vi "Retrieve trace.vi"(5 "max points":i32, 6 "error in (no error)":errorcluster, 7 "Data.PG in":refnum<class "Data.PG.lvclass">, 8 "Column path":string, 9 "Table path":string, 10 "End":timestamp, 11 "Start":timestamp) -> (0 "error out":errorcluster, 2 "Trace":cluster{timestamp[], dbl[]}, 3 "Data.PG out":refnum<class "Data.PG.lvclass">)   [LabVIEW 2020, in "Data.PG.lvclass"]
uses:
  Data.PG.lvclass
  <vilib>/Utility/error.llb/Error Cluster From Error Code.vi
  <vilib>/ErrorRing/Error Ring.xnode
panel:
  out "resulting string":string
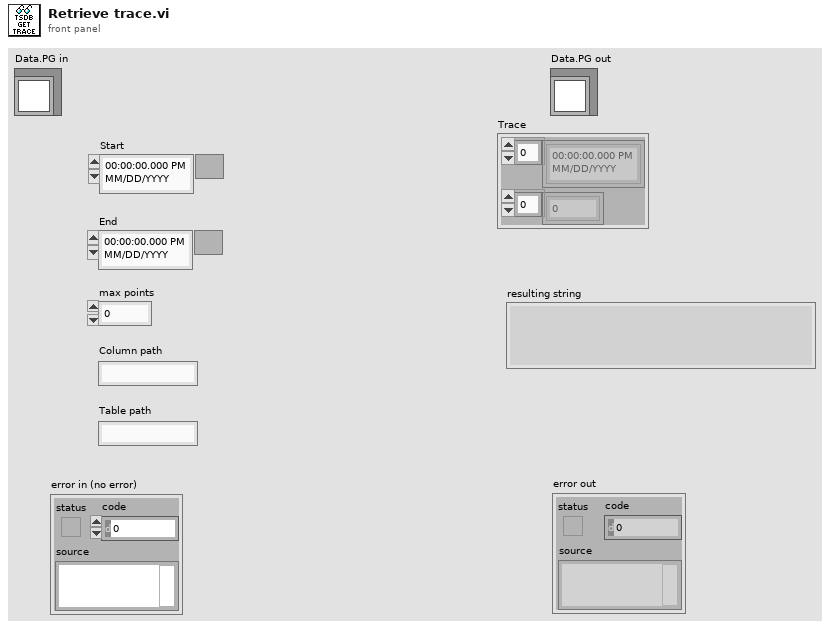
[diagram p1: front panel]
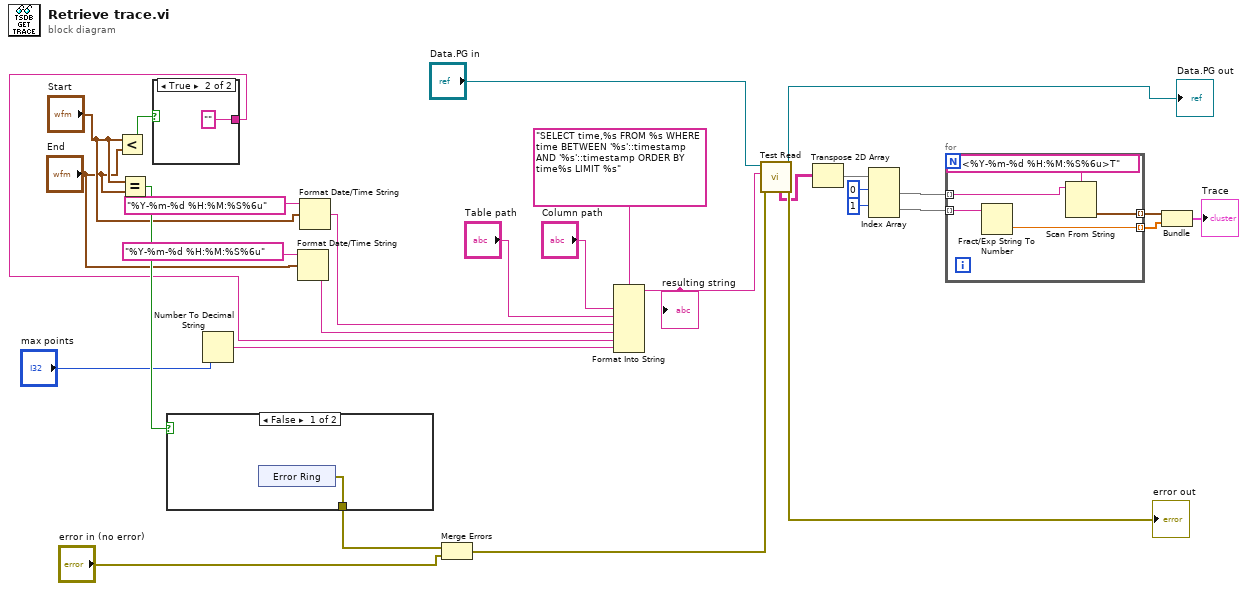
[diagram p0: block diagram]
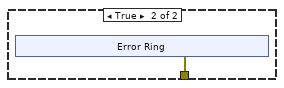
[diagram p2: hidden frame]
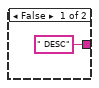
[diagram p3: hidden frame]
diagram:
  n1 = Less?(x="Start", y="End") -> (x < y?=w27:bool)
  n2 = Equal?(x="Start", y="End") -> (x = y?=w26:bool)
  n3 = case shown="True" w27 {
    tunnel: [" DESC" ""] -> w1
    frame False {
    }
    frame True {
    }
  }
  n4 = case shown="False" w26 {
    tunnel: [w33 w35] -> w25
    frame False {
      n5 = xnode "Error Ring"() -> ("error out"=w33:errorcluster)
    }
    frame True {
      n6 = xnode "Error Ring"() -> ("error out"=w35:errorcluster)
    }
  }
  n7 = Number To Decimal String(number="max points") -> (decimal integer string=w2:string)  [unwired: 1 in]
  n8 = Format Date/Time String(time format string (%c)="%Y-%m-%d %H:%M:%S%6u", seconds (now)="End") -> (date/time string=w5:string)  [unwired: 1 in]
  n9 = Format Date/Time String(time format string (%c)="%Y-%m-%d %H:%M:%S%6u", seconds (now)="Start") -> (date/time string=w6:string)  [unwired: 1 in]
  n10 = Merge Errors(w25, "error in (no error)") -> (w23:errorcluster)
  n11 = Format Into String(format string="SELECT time,%s FROM %s WHERE time BETWEEN '%s'::timestamp AND '%s'::timestamp ORDER BY time%s LIMIT %s", "Column path", "Table path", w6, w5, w1, w2) -> (resulting string=w3:string)  [unwired: 2 in, 1 out]
  "resulting string" <- w3
  n12 = call-dynamic "Test Read.vi"("error in (no error)"=w23, "command"=w3, "Data.PG in"="Data.PG in") -> ("error out"=→"error out":errorcluster, "Data.PG out"=→"Data.PG out":refnum<class "Data.PG.lvclass">, "Result"=w22:string[][])  [unwired: 3 in, 3 out]
  n13 = Transpose 2D Array(2D array=w22) -> (transposed array=w21:string[][])
  n14 = Index Array(array=w21, index (row) #1=0 ("index (row)"), index (row) #2=1 ("index (row)")) -> (element #1=w18:string[], element #2=w17:string[])  [unwired: 2 in]
  n15 = for {
    tunnel: w18 -> [w44] mode=indexing
    tunnel: w17 -> [w43] mode=indexing
    tunnel: [w42] -> w15 mode=indexing
    tunnel: [w41] -> w16 mode=indexing
    n16 = Fract/Exp String To Number(string=w43) -> (number=w42:dbl)  [unwired: 3 in, 1 out]
    n17 = Scan From String(format string="%<%Y-%m-%d %H:%M:%S%6u>T", input string=w44) -> (output 1=w41:timestamp)  [unwired: 3 in, 3 out]
  }
  n18 = Bundle(w16, w15) -> (→"Trace":cluster{timestamp[], dbl[]})  [unwired: 1 in]
